vi "CRYRun Preprocessing.vi"(0 "Type A":enum16{"Curves", "Values", "Results", "WFM"}(ring), 1 "user equation cluster":T1 {"Results axis" items=["x", "y", "z"]; "Input axis" items=["x", "y", "z"]; "Custom unit results array"."dB ref" format="%.2f"; "Custom unit input array"."dB ref" format="%.2f"}, 2 "No.VI":i32, 5 "Type B":enum16{"Curves", "Values", "Results", "WFM"}(ring), 7 "Type":u16(ring) items=["Arithmetic", "Constant", "Unary", "Scalar(Statistics)", "Smoothing", "Intersection(Search)", "User Equation", "Windowing", "Resolution", "Directivity Index", "1/n Octave Synthesis", "Resampling", "Frequency Shift"], 9 "Binary Operator":u16(ring) items=["+", "--", "x", "÷"], 11 "Work in":u16(slide), 12 "Unary Operator":u16(ring) items=["Change Sign", "Reciprocal Value", "Absolute Value", "Square", "Square Root", "Exp", "Ln", "Unwarp Phase", "Group Delay", "FFT", "Inverse FFT"], 13 "Statistical Operator":u16(ring) items=["Average", "Power Sum", "Maximum", "Minimum", "Est. Resonance", "Est. Notch", "IEEE TOLP", "IEEE ROLP", "IEEE SOLP", "ITU-T SLR", "ITU-T RLR", "ITU-T RLR w/Leak", "ITU-T STMR", "Attack Time", "Release Time", "Zwicker Loudness"], 14 "Result Data":string[](array[string])) -> (4 "Run Flag":bool, 6 "Message Mode":u16, 8 "Invalid Variable":string[](array[string]), 10 "index of Invalid":i32)   [LabVIEW 2013]
uses:
  Typedef Control/CRYUser Equation Cluster.ctl
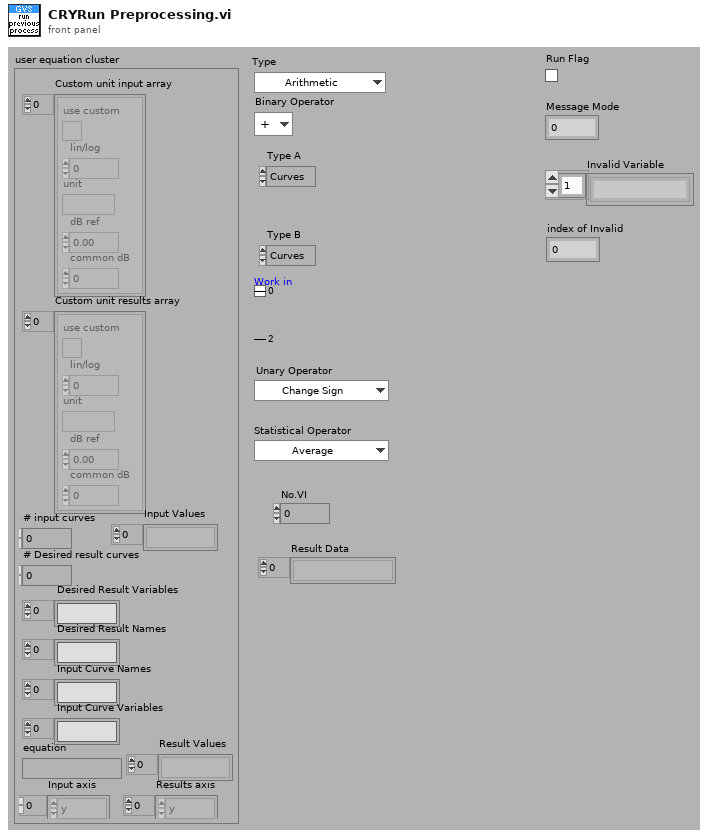
[diagram p1: front panel]
types:
  T1 = typedef "CRYUser Equation Cluster.ctl" = cluster{"Custom unit input array":cluster{"use custom":bool, "lin/log":u16, "unit":string, "dB ref":dbl, "common dB":u16}[], "Custom unit results array ":cluster{"use custom":bool, "lin/log":u16, "unit":string, "dB ref":dbl, "common dB":u16}[], "Desired Result Variables":string[], "Desired Result Names":string[], "Input Curve Names":string[], "Input Curve Variables":string[], "equation":string, "Input axis":u16[], "Results axis":u16[], "# input curves":i32, "# Desired result curves ":i32, "Input Values":string[], "Result Values":string[]}
  T2 = typedef "CRYData Cluster Array.ctl" = T3[]
  T3 = typedef "CRYData Cluster.ctl" = cluster{"Name":string, "Curve":cluster{"x":dbl, "y":dbl, "z":dbl}[], "X data":u16, "Y data":u16, "Z data":u16, "X axis":u16, "Y axis":u16, "Z axis":u16, "X unit":string, "Y unit":string, "Z unit":string, "X dB ref":dbl, "Y dB ref":dbl, "Z dB ref":dbl, "single val":bool, "protected":bool, "display X":bool, "display Y":bool, "display Z":bool, "Test Info":string, "Step No.":i32, "Plot Settings":cluster{"Color":u32, "Interpolation":u8, "Point Style":u8, "Line Style":u8, "Point Color":u32, "Line Width":u8, "Bar Plot Style":u8, "Fill To":i16}, "AutoProtect":bool}
  T4 = typedef "CRYWaveform Cluster Array.ctl" = T5[]
  T5 = typedef "CRYWaveform Cluster.ctl" = cluster{"Waveform":cluster{"X0":dbl, "dX":dbl, "Y":sgl[]}, "X data":u16, "Y data":u16, "Y axis":u16, "X unit":string, "Y unit":string, "Y dB ref":dbl, "display Y":bool, "display X":bool, "Overload?":bool, "Test Info":string, "Step No.":i32, "Name":string, "protected":bool, "Sqc history":string[], "Signal Channel ID":i32, "Plot Settings":cluster{"Color":u32, "Interpolation":u8, "Point Style":u8, "Line Style":u8, "Point Color":u32, "Line Width":u8, "Bar Plot Style":u8, "Fill To":i16}, "AutoProtect":bool}
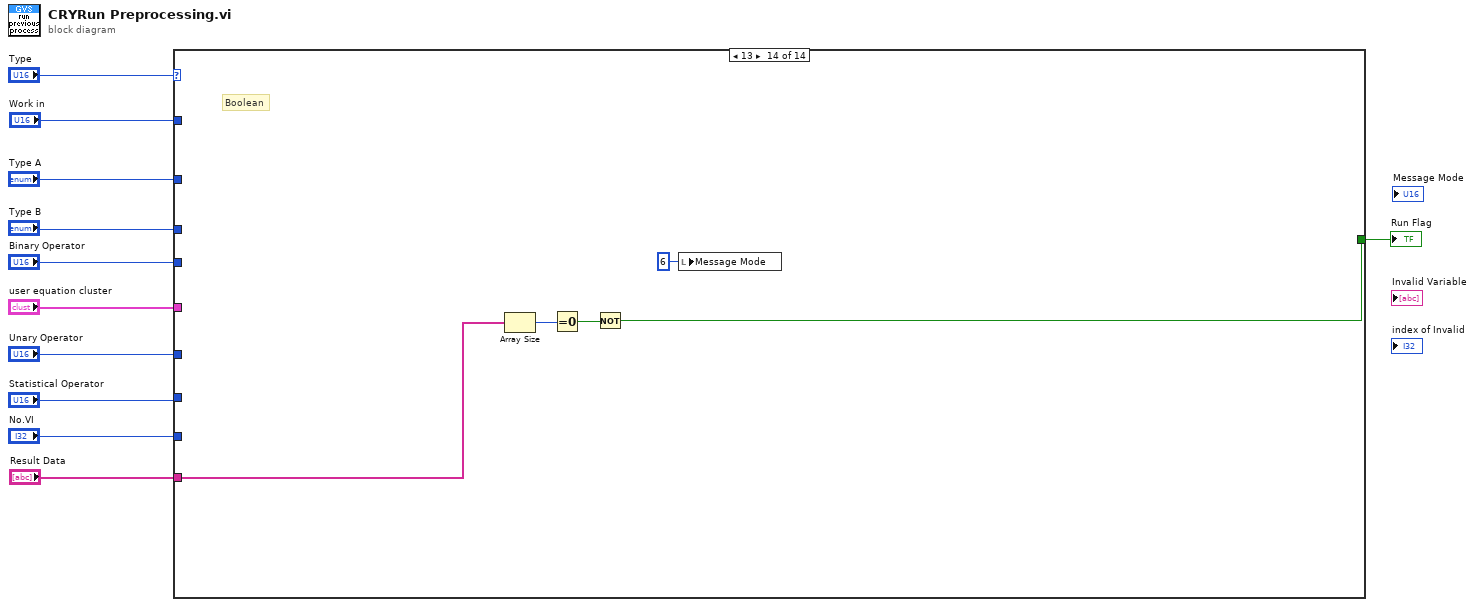
[diagram p0: block diagram]
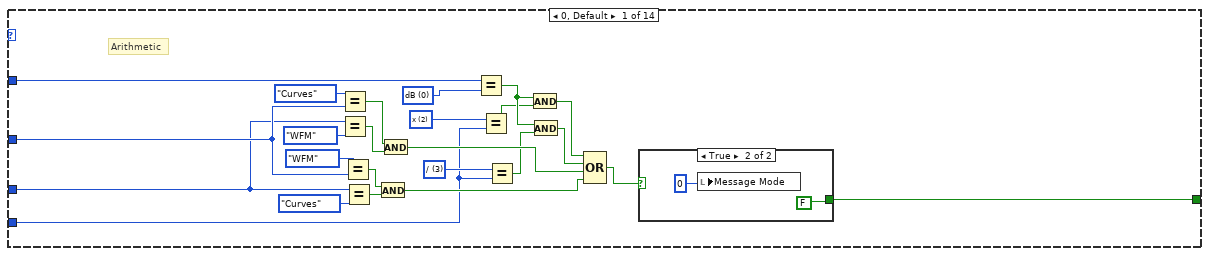
[diagram p2: hidden frame]
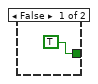
[diagram p3: hidden frame]
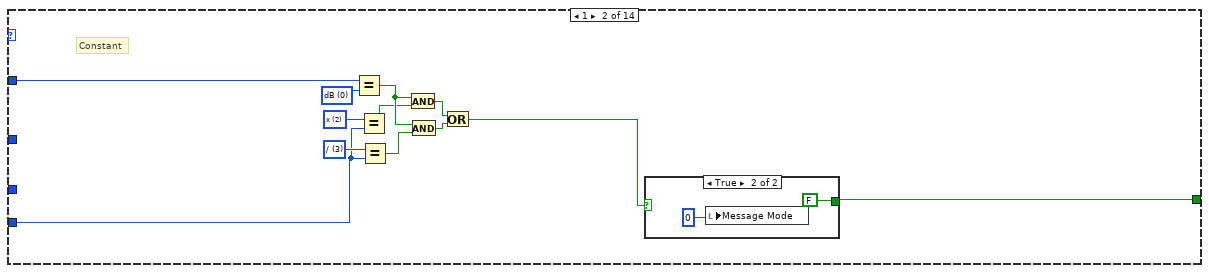
[diagram p4: hidden frame]
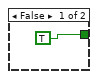
[diagram p5: hidden frame]
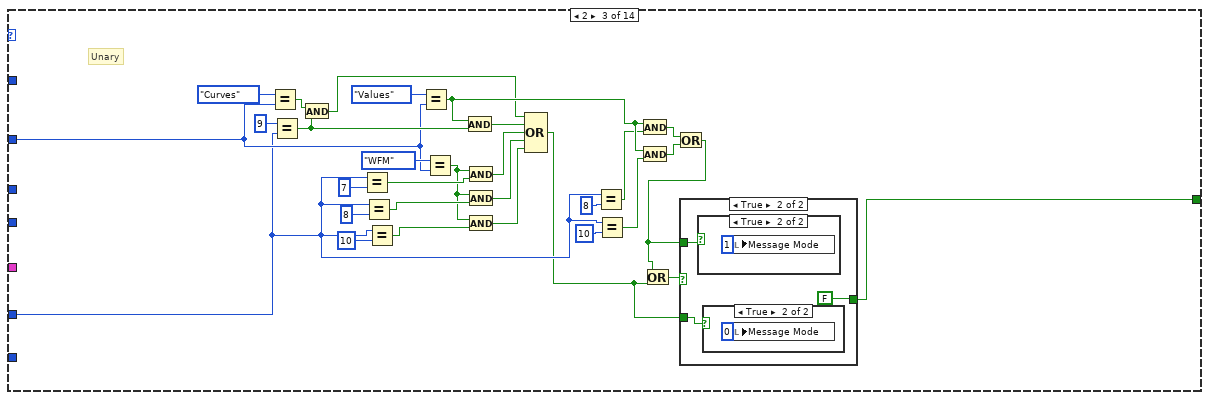
[diagram p6: hidden frame]
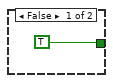
[diagram p7: hidden frame]
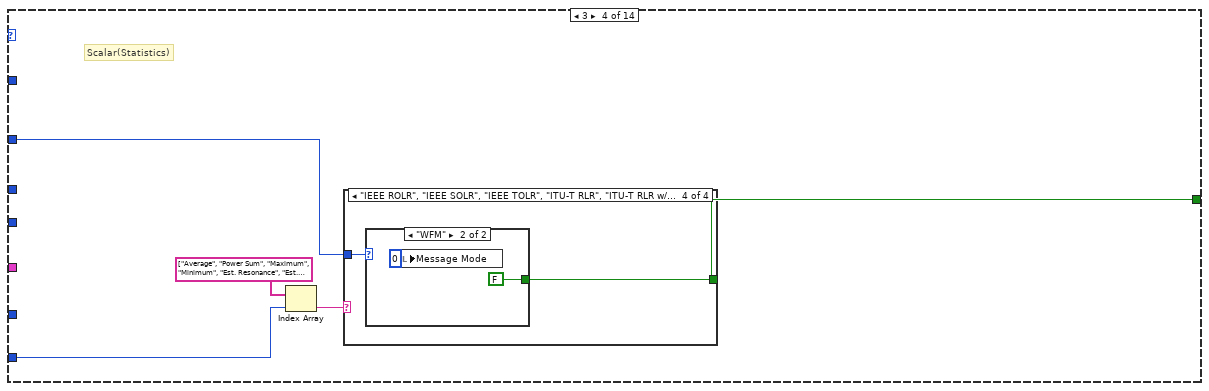
[diagram p10: hidden frame]
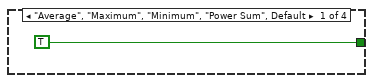
[diagram p11: hidden frame]
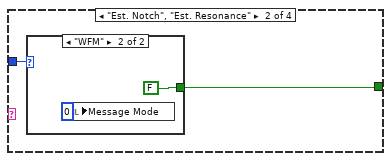
[diagram p12: hidden frame]
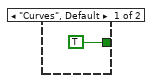
[diagram p13: hidden frame]
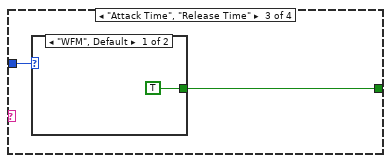
[diagram p14: hidden frame]
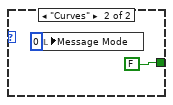
[diagram p15: hidden frame]
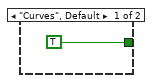
[diagram p16: hidden frame]
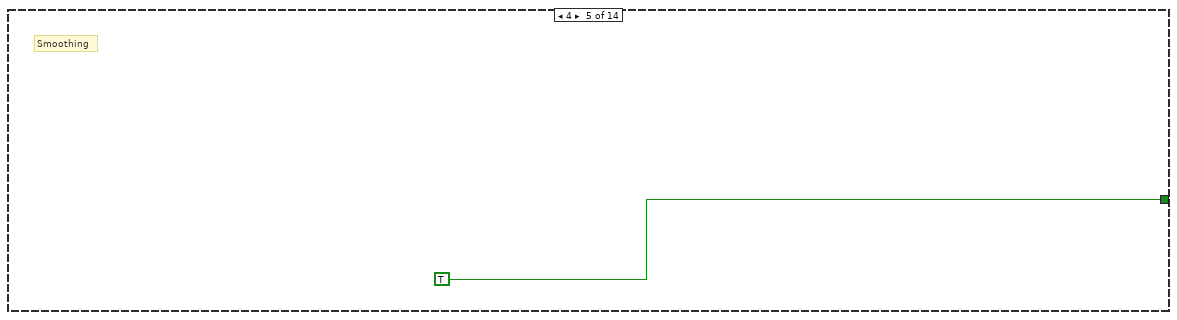
[diagram p17: hidden frame]
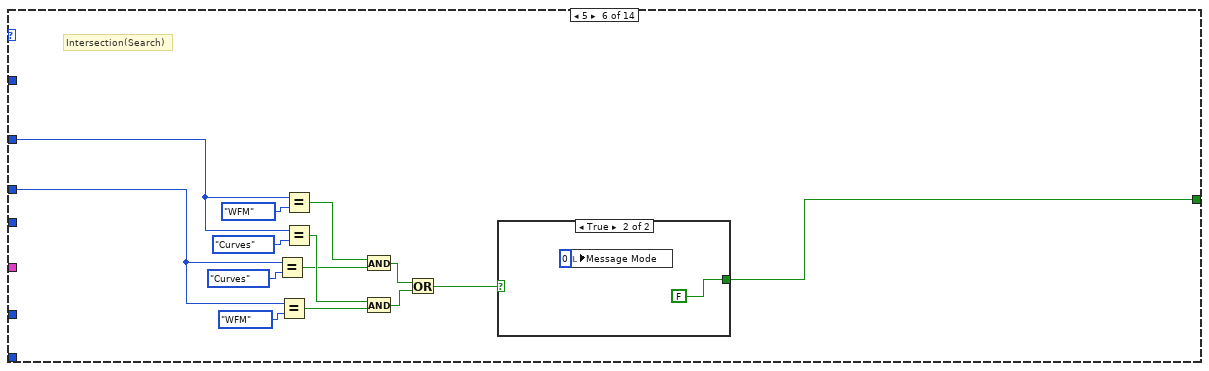
[diagram p18: hidden frame]
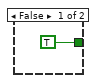
[diagram p19: hidden frame]
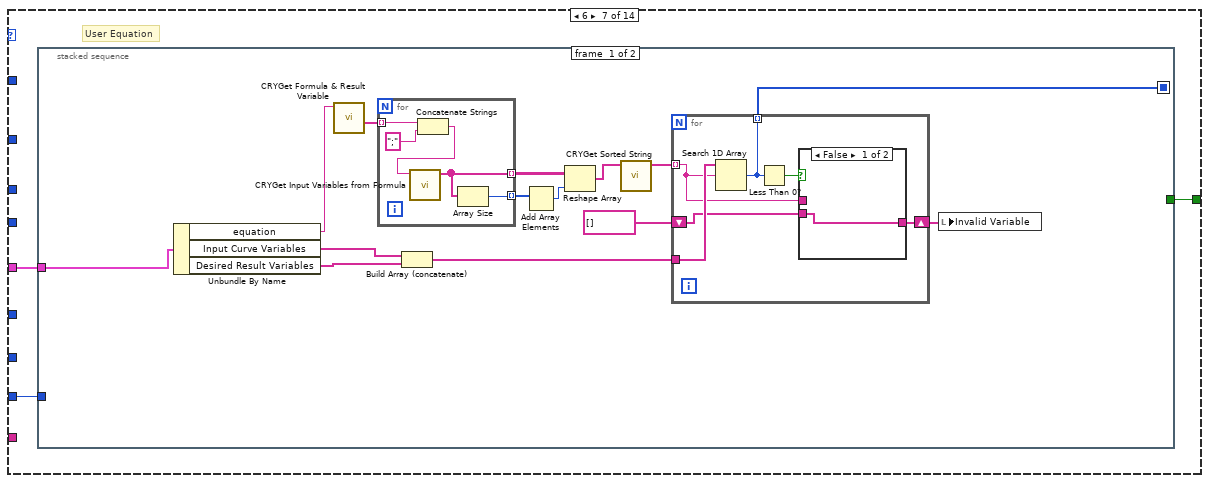
[diagram p20: hidden frame]
diagram:
  n1 = case shown="13" "Type" {
    tunnel: "Type A" -> [w15 _ w59 w95 _ w117 _ _ _ _ _ _ _ _]
    tunnel: "Type B" -> [w14 _ _ _ _ w114 _ _ _ _ _ _ _ _]
    tunnel: "Work in" -> [w17 w42 _ _ _ _ _ _ _ _ _ _ _ _]
    tunnel: [w12 w39 w56 w93 TRUE w119 w132 TRUE TRUE TRUE TRUE w218 w224 w232] -> w11
    tunnel: "Unary Operator" -> [_ _ w58 _ _ _ _ _ _ _ _ _ _ _]
    tunnel: "Statistical Operator" -> [_ _ _ w91 _ _ _ _ _ _ _ _ _ _]
    tunnel: "Binary Operator" -> [w16 w41 _ _ _ _ _ _ _ _ _ _ _ _]
    tunnel: "user equation cluster" -> [_ _ _ _ _ _ w131 _ _ _ _ _ _ _]
    tunnel: "No.VI" -> [_ _ _ _ _ _ w130 _ _ _ _ w222 w225 _]
    tunnel: "Result Data" -> [_ _ _ _ _ _ _ _ _ _ _ _ _ w231]
    frame 0, Default {
      w29 = u16 3 items=["+", "--", "x", "/"] ("Operator")
      w27 = u16 2 items=["+", "--", "x", "/"] ("Operator")
      w26 = u16 0 items=["dB", "Linear", "Power"] ("Work in")
      # "Arithmetic"
      n2 = Equal?(x=enum16{"Curves", "Values", "Results", "WFM"}."Curves" ("Type A"), y=w15) -> (x = y?=w20:bool)
      n3 = Equal?(x=w14, y=enum16{"Curves", "Values", "Results", "WFM"}."WFM") -> (x = y?=w21:bool)
      n4 = Equal?(x=enum16{"Curves", "Values", "Results", "WFM"}."WFM" ("Type A"), y=w15) -> (x = y?=w24:bool)
      n5 = Equal?(x=w14, y=enum16{"Curves", "Values", "Results", "WFM"}."Curves") -> (x = y?=w25:bool)
      n6 = And(x=w24, y=w25) -> (x .and. y?=w35:bool)
      n7 = And(x=w20, y=w21) -> (x .and. y?=w34:bool)
      n8 = Equal?(x=w17, y=w26) -> (x = y?=w30:bool)
      n9 = Equal?(x=w27, y=w16) -> (x = y?=w28:bool)
      n10 = Equal?(x=w29, y=w16) -> (x = y?=w31:bool)
      n11 = And(x=w30, y=w28) -> (x .and. y?=w32:bool)
      n12 = And(x=w30, y=w31) -> (x .and. y?=w33:bool)
      n13 = Compound Arithmetic op=OR(w32, w33, w34, w35) -> (w13:bool)
      n14 = case shown="True" w13 {
        tunnel: [TRUE FALSE] -> w12
        frame False {
        }
        frame True {
          n15 = local write "Message Mode"(u16 0 ("Message Mode")) -> ()
        }
      }
    }
    frame 1 {
      w46 = u16 3 items=["+", "--", "x", "/"] ("Operator")
      w44 = u16 2 items=["+", "--", "x", "/"] ("Operator")
      w43 = u16 0 items=["dB", "Linear", "Power"] ("Work in")
      # "Constant"
      n16 = Equal?(x=w42, y=w43) -> (x = y?=w47:bool)
      n17 = Equal?(x=w44, y=w41) -> (x = y?=w45:bool)
      n18 = Equal?(x=w46, y=w41) -> (x = y?=w48:bool)
      n19 = And(x=w47, y=w45) -> (x .and. y?=w50:bool)
      n20 = And(x=w47, y=w48) -> (x .and. y?=w49:bool)
      n21 = Or(x=w50, y=w49) -> (x .or. y?=w40:bool)
      n22 = case shown="True" w40 {
        tunnel: [TRUE FALSE] -> w39
        frame False {
        }
        frame True {
          n23 = local write "Message Mode"(u16 0 ("Message Mode")) -> ()
        }
      }
    }
    frame 2 {
      # "Unary"
      n24 = Equal?(x=enum16{"Curves", "Values", "Results", "WFM"}."Curves", y=w59) -> (x = y?=w62:bool)
      n25 = Equal?(x=u16 9, y=w58) -> (x = y?=w64:bool)
      n26 = And(x=w62, y=w64) -> (x .and. y?=w73:bool)
      n27 = Equal?(x=w58, y=u16 7) -> (x = y?=w70:bool)
      n28 = Equal?(x=w58, y=u16 8) -> (x = y?=w71:bool)
      n29 = Equal?(x=w58, y=u16 10) -> (x = y?=w72:bool)
      n30 = Equal?(x=enum16{"Curves", "Values", "Results", "WFM"}."Values", y=w59) -> (x = y?=w81:bool)
      n31 = Equal?(x=enum16{"Curves", "Values", "Results", "WFM"}."WFM", y=w59) -> (x = y?=w69:bool)
      n32 = And(x=w81, y=w64) -> (x .and. y?=w74:bool)
      n33 = And(x=w69, y=w70) -> (x .and. y?=w75:bool)
      n34 = And(x=w69, y=w71) -> (x .and. y?=w76:bool)
      n35 = And(x=w69, y=w72) -> (x .and. y?=w77:bool)
      n36 = Compound Arithmetic op=OR(w73, w74, w75, w76, w77) -> (w54:bool)
      n37 = Equal?(x=w58, y=u16 8) -> (x = y?=w80:bool)
      n38 = Equal?(x=w58, y=u16 10) -> (x = y?=w82:bool)
      n39 = And(x=w81, y=w80) -> (x .and. y?=w83:bool)
      n40 = And(x=w81, y=w82) -> (x .and. y?=w84:bool)
      n41 = Or(x=w83, y=w84) -> (x .or. y?=w55:bool)
      n42 = Or(x=w55, y=w54) -> (x .or. y?=w57:bool)
      n43 = case shown="True" w57 {
        tunnel: [TRUE FALSE] -> w56
        tunnel: w55 -> [_ w87]
        tunnel: w54 -> [_ w86]
        frame False {
        }
        frame True {
          n44 = case shown="True" w87 {
            frame False {
            }
            frame True {
              n45 = local write "Message Mode"(u16 1 ("Message Mode")) -> ()
            }
          }
          n46 = case shown="True" w86 {
            frame False {
            }
            frame True {
              n47 = local write "Message Mode"(u16 0 ("Message Mode")) -> ()
            }
          }
        }
      }
    }
    frame 3 {
      # "Scalar(Statistics)"
      n48 = Index Array(array=string[] ["Average", "Power Sum", "Maximum", "Minimum", "Est. Resonance", "Est. Notch", "IEEE TOLR", "IEEE ROLR", "IEEE SOLR", "ITU-T SLR", "ITU-T RLR", "ITU-T RLR w/ Leak", "ITU-T STMR", "Attack Time", "Release Time", "Zwicker"] ("Scalar Op Name"), index=w91) -> (element=w94:string)
      n49 = case shown="\"IEEE ROLR\", \"IEEE SOLR\", \"IEEE TOLR\", \"ITU-T RLR\", \"ITU-T RLR w/ Leak\", \"ITU-T SLR\", \"ITU-T STMR\", \"Zwicker\"" w94 {
        tunnel: w95 -> [_ w98 w103 w108]
        tunnel: [TRUE w97 w102 w107] -> w93
        frame "Average", "Maximum", "Minimum", "Power Sum", Default {
        }
        frame "Est. Notch", "Est. Resonance" {
          n50 = case shown="\"WFM\"" w98 {
            tunnel: [TRUE FALSE ("x")] -> w97
            frame "Curves", Default {
            }
            frame "WFM" {
              n51 = local write "Message Mode"(u16 0 ("Message Mode")) -> ()
            }
          }
        }
        frame "Attack Time", "Release Time" {
          n52 = case shown="\"WFM\", Default" w103 {
            tunnel: [TRUE FALSE] -> w102
            frame "WFM", Default {
            }
            frame "Curves" {
              n53 = local write "Message Mode"(u16 0 ("Message Mode")) -> ()
            }
          }
        }
        frame "IEEE ROLR", "IEEE SOLR", "IEEE TOLR", "ITU-T RLR", "ITU-T RLR w/ Leak", "ITU-T SLR", "ITU-T STMR", "Zwicker" {
          n54 = case shown="\"WFM\"" w108 {
            tunnel: [TRUE FALSE] -> w107
            frame "Curves", Default {
            }
            frame "WFM" {
              n55 = local write "Message Mode"(u16 0 ("Message Mode")) -> ()
            }
          }
        }
      }
    }
    frame 4 {
      # "Smoothing"
    }
    frame 5 {
      # "Intersection(Search)"
      n56 = Equal?(x=w114, y=enum16{"Curves", "Values", "Results", "WFM"}."Curves" ("Type A")) -> (x = y?=w113:bool)
      n57 = Equal?(x=w114, y=enum16{"Curves", "Values", "Results", "WFM"}."WFM" ("Type A")) -> (x = y?=w126:bool)
      n58 = Equal?(x=w117, y=enum16{"Curves", "Values", "Results", "WFM"}."WFM" ("Type A")) -> (x = y?=w125:bool)
      n59 = Equal?(x=w117, y=enum16{"Curves", "Values", "Results", "WFM"}."Curves" ("Type A")) -> (x = y?=w116:bool)
      n60 = And(x=w125, y=w113) -> (x .and. y?=w123:bool)
      n61 = And(x=w116, y=w126) -> (x .and. y?=w124:bool)
      n62 = Or(x=w123, y=w124) -> (x .or. y?=w120:bool)
      n63 = case shown="True" w120 {
        tunnel: [TRUE FALSE] -> w119
        frame False {
        }
        frame True {
          n64 = local write "Message Mode"(u16 0 ("Message Mode")) -> ()
        }
      }
    }
    frame 6 {
      # "User Equation"
      n65 = stacked-sequence {
        seq-local: [w138 _] -> [_ w172]
        tunnel: [_ w173] -> w132
        tunnel: w131 -> [w146 w171]
        tunnel: w130 -> [_ w162]
        frame #0 {
          n66 = Unbundle By Name(w146) -> ("equation"=w145:string, "Input Curve Variables"=w137:string[], "Desired Result Variables"=w135:string[])
          n67 = call "CRYGet Formula & Result Variable.vi"("String"=w145) -> ("Formula Out"=w144:string[])  [unwired: 8 in, 2 out]
          n68 = for {
            tunnel: w144 -> [w159] mode=indexing
            tunnel: [w161] -> w143 mode=indexing
            tunnel: [w160] -> w140 mode=indexing
            n69 = Concatenate Strings(w159, ";" ("string")) -> (w157:string)
            n70 = call "CRYGet Input Variables from Formula.vi"("Formula string"=w157) -> ("Variables Out"=w161:string[])  [unwired: 10 in]
            n71 = Array Size(array=w161) -> (size(s)=w160:i32)
          }
          n72 = Build Array (concatenate)(w137, w135) -> (w136:string[])
          n73 = Add Array Elements(numeric array=w140) -> (sum=w141:i32)
          n74 = Reshape Array(w143, w141) -> (w142:string[])
          n75 = call "CRYGet Sorted String.vi"("Variables In"=w142) -> ("Variables Out"=w139:string[])  [unwired: 10 in]
          n76 = for {
            tunnel: w139 -> [w150] mode=indexing
            tunnel: w136 -> [w152]
            tunnel: [w149] -> w138 mode=indexing
            shift-right: [w147] -> w133
            shift-left: string[] [] ("Variables Out") -> [w148]
            n77 = Search 1D Array(1D array=w152, element=w150) -> (index of element=w149:i32)  [unwired: 1 in]
            n78 = Less Than 0?(x=w149) -> (x < 0?=w151:bool)
            n79 = case shown="False" w151 {
              tunnel: w150 -> [_ w155]
              tunnel: w148 -> [w153 w156]
              tunnel: [w153 w154] -> w147
              frame False {
              }
              frame True {
                n80 = Insert Into Array(array=w156, new element=w155) -> (w154:string[])  [unwired: 1 in]
              }
            }
          }
          n81 = local write "Invalid Variable"(w133) -> ()
        }
        frame #1 {
          n82 = local read "Invalid Variable"() -> (w174:string[])
          n83 = Unbundle By Name(w171) -> ("Input Curve Names"=w167:string[])
          n84 = call "CRYGet Upper Step Data.vi"("Type In"=enum16{"Curves", "Values", "Results", "WFM"}."Curves", "No.VI"=w162) -> ("Curve array"=w164:T2)  [unwired: 9 out]
          n85 = call "CRYGet Upper Step Data.vi"("Type In"=enum16{"Curves", "Values", "Results", "WFM"}."Values", "No.VI"=w162) -> ("Value array"=w163:T2)  [unwired: 9 out]
          n86 = Array Size(array=w174) -> (size(s)=w176:i32)
          n87 = Build Array (concatenate)(w164, w163) -> (w169:T2)
          n88 = Equal To 0?(x=w176) -> (x = 0?=w175:bool)
          n89 = Array Size(array=w167) -> (size(s)=w168:i32)
          n90 = case shown="True" w175 {
            tunnel: [FALSE w186] -> w173
            tunnel: w172 -> [_ w192]
            tunnel: w167 -> [_ w183]
            tunnel: "User Defined Constant" -> [_ w191]
            tunnel: w169 -> [_ w190]
            tunnel: w168 -> [_ w184]
            frame False {
              n91 = local write "Message Mode"(u16 2 ("Message Mode")) -> ()
            }
            frame True {
              n92 = for {
                tunnel: w192 -> [w202] mode=indexing
                tunnel: w183 -> [w211]
                tunnel: w191 -> [w210]
                tunnel: w190 -> [w209]
                tunnel: [w203] -> w189 mode=indexing
                tunnel: [w202] -> w182
                tunnel: w184 -> [w201]
                stop <- w203 continue-if-true
                n93 = for {
                  tunnel: w209 -> [w213] mode=indexing
                  tunnel: [w212] -> w207 mode=indexing
                  n94 = Unbundle By Name(w213) -> ("Name"=w212:string)
                }
                n95 = Greater Or Equal?(x=w202, y=w201) -> (x >= y?=w200:bool)
                n96 = Index Array(array=w211, index=w202) -> (element=w208:string)
                n97 = Equal?(x=w208, y=w210) -> (x = y?=w204:bool)
                n98 = Search 1D Array(1D array=w207, element=w208) -> (index of element=w206:i32)  [unwired: 1 in]
                n99 = Greater Or Equal To 0?(x=w206) -> (x >= 0?=w205:bool)
                n100 = Compound Arithmetic op=OR(w200, w205, w204) -> (w203:bool)
              }
              n101 = Index Array(array=w183, index=w182) -> (element=w181:string)
              n102 = Search 1D Array(1D array=w189, element=FALSE) -> (index of element=w185:i32)  [unwired: 1 in]
              n103 = Less Than 0?(x=w185) -> (x < 0?=w187:bool)
              n104 = Equal?(x="<Select Operand>", y=w181) -> (x = y?=w179:bool)
              n105 = case shown="False" w187 {
                selector: w187 -> [w194 w199]
                tunnel: [w194 w199] -> w186
                tunnel: w182 -> [w195 _]
                tunnel: w179 -> [w193 _]
                frame False {
                  n106 = case shown="True" w193 {
                    tunnel: w195 -> [w197 _]
                    frame False {
                      n107 = local write "index of Invalid"(w197) -> ()
                      n108 = local write "Message Mode"(u16 3 ("Message Mode")) -> ()
                    }
                    frame True {
                      n109 = local write "Message Mode"(u16 4 ("Message Mode")) -> ()
                    }
                  }
                }
                frame True {
                }
              }
            }
          }
        }
      }
    }
    frame 7 {
      # "Windowing"
    }
    frame 8 {
      # "Resolution"
    }
    frame 9 {
      # "Directivity Index"
    }
    frame 10 {
      # "1/n Octave Synthesis"
    }
    frame 11 {
      # "Resampling"
      n110 = call "CRYGet Upper Step Data.vi"("Type In"=enum16{"Curves", "Values", "Results", "WFM"}."WFM", "No.VI"=w222) -> ("Waveform Array"=w221:T4)  [unwired: 9 out]
      n111 = Array Size(array=w221) -> (size(s)=w220:i32)
      n112 = Equal To 0?(x=w220) -> (x = 0?=w219:bool)
      n113 = Not(x=w219) -> (.not. x?=w218:bool)
    }
    frame 12 {
      # "Frequency Shift"
      n114 = call "CRYGet Upper Step Data.vi"("Type In"=enum16{"Curves", "Values", "Results", "WFM"}."WFM", "No.VI"=w225) -> ("Waveform Array"=w228:T4)  [unwired: 9 out]
      n115 = Array Size(array=w228) -> (size(s)=w227:i32)
      n116 = Equal To 0?(x=w227) -> (x = 0?=w226:bool)
      n117 = Not(x=w226) -> (.not. x?=w224:bool)
    }
    frame 13 {
      # "Boolean"
      n118 = Array Size(array=w231) -> (size(s)=w234:i32)
      n119 = Equal To 0?(x=w234) -> (x = 0?=w233:bool)
      n120 = Not(x=w233) -> (.not. x?=w232:bool)
      n121 = local write "Message Mode"(u16 6 ("Message Mode")) -> ()
    }
  }
  "Run Flag" <- w11
